vi "VPA QC Update Flow Data.vi"(7 "Density of Fluid":dbl, 8 "Flow Rate Test Data":T1, 9 "Digital \nScale Read":refnum<vi>, 11 "Set":bool) -> (0 "Rate Data Out":T1, 1 "% Difference":dbl, 2 "Flow Rate":dbl, 3 "Calculated Volume":dbl)   [LabVIEW 2013]
uses:
  Controls/VPA QC Flow Rate Data Cluster.ctl
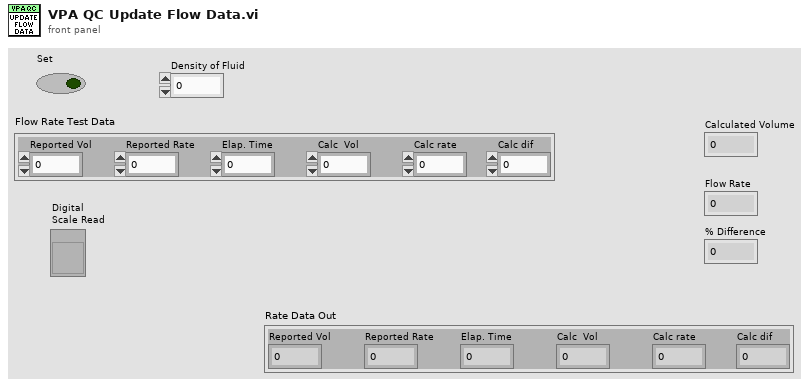
[diagram p1: front panel]
types:
  T1 = typedef "VPA QC Flow Rate Data Cluster.ctl" = cluster{"Reported Vol":dbl, "Reported Rate":dbl, "Elap. Time":dbl, "Calc  Vol":dbl, "Calc rate":dbl, "Calc dif":dbl}
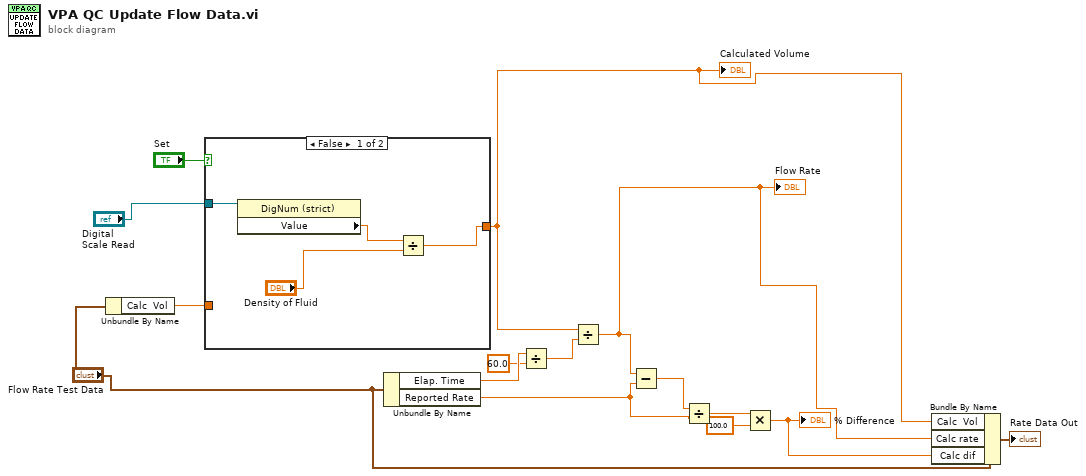
[diagram p0: block diagram]
diagram:
  n1 = Unbundle By Name("Flow Rate Test Data") -> ("Calc  Vol"=w14:dbl)
  n2 = case shown="False" "Set" {
    tunnel: "Digital \nScale Read" -> [w19 _]
    tunnel: w14 -> [_ w20]
    tunnel: [w16 w20] -> w4
    frame False {
      n3 = property class="DigNum (strict)"(reference=w19) -> ("Value"=w18:dbl)  [unwired: 1 in, 2 out]
      n4 = Divide(x=w18, y="Density of Fluid") -> (x/y=w16:dbl)
    }
    frame True {
    }
  }
  "Calculated Volume" <- w4
  n5 = Unbundle By Name("Flow Rate Test Data") -> ("Elap. Time"=w12:dbl, "Reported Rate"=w8:dbl)
  n6 = Divide(x=w12, y=60.0) -> (x/y=w10:dbl)
  n7 = Divide(x=w4, y=w10) -> (x/y=w3:dbl)
  "Flow Rate" <- w3
  n8 = Subtract(x=w3, y=w8) -> (x-y=w9:dbl)
  n9 = Divide(x=w9, y=w8) -> (x/y=w7:dbl)
  n10 = Multiply(x=w7, y=100.0) -> (x*y=w2:dbl)
  "% Difference" <- w2
  n11 = Bundle By Name(cluster="Flow Rate Test Data", "Calc  Vol"=w4, "Calc rate"=w3, "Calc dif"=w2) -> (→"Rate Data Out":T1)
